vi "Switch Configure (3706).vi"(7 "Resistivity":T1, 8 "error in (no error)":errorcluster, 11 "VISA resource name in":refnum<visa-resource-name>) -> (0 "error out":errorcluster, 3 "VISA resource name out":refnum<visa-resource-name>)   [LabVIEW 2016, in "Hall Effect Library.lvlib"]
uses:
  Hall Effect Library.lvlib
  Public/Controls/Resisitivity.ctl
  Global Variables/Test Settings.vi
  <instrlib>/Keithley 3706/Keithley 3706.lvlib
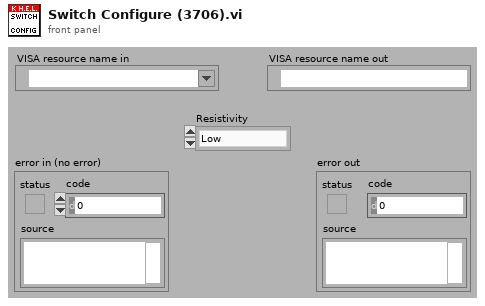
[diagram p1: front panel]
types:
  T1 = typedef "Hall Effect Library.lvlib/Resisitivity.ctl" = enum16{"Low", "High"}
  T2 = enum16{"BBM:Break Before Make", "MBB:Make Before Break", "OFF"}
  T3 = enum16{"None", "7052", "7053", "7054", "7056", "7057", "7058", "7059", "7061", "7062", "7063", "7064", "7065", "7066", "7067", "7152", "7153", "7154", "7156", "7158", "7164", "7166", "7168", "7169", "7402", "9990", "9991"}
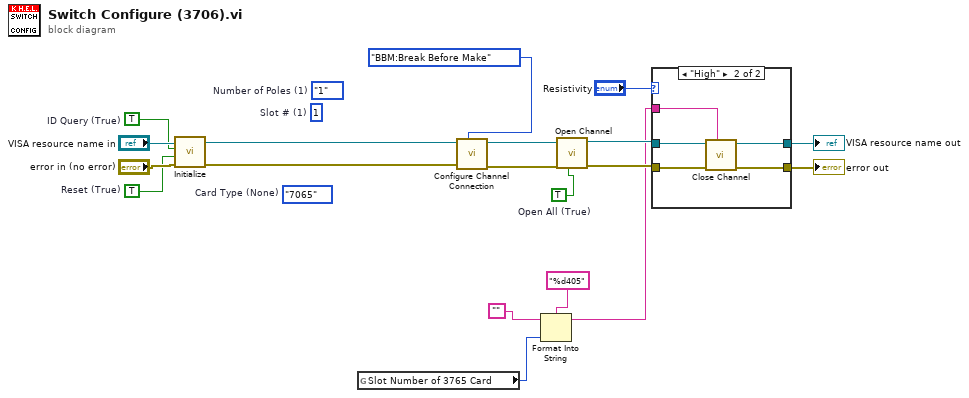
[diagram p0: block diagram]
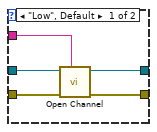
[diagram p2: hidden frame]
diagram:
  w9 = TRUE  # Open All (True)
  (unwired) enum16{"1", "2", "4"}."1"  # Number of Poles (1)
  (unwired) T3."7065"  # Card Type (None)
  w14 = TRUE  # Reset (True)
  w13 = TRUE  # ID Query (True)
  (unwired) u32 1  # Slot # (1)
  n1 = call <instrlib>:"Initialize.vi"("error in (no error)"="error in (no error)", "Reset (True)"=w14, "ID Query (True)"=w13, "VISA resource name"="VISA resource name in") -> ("error out"=w11:errorcluster, "VISA resource name out"=w12:refnum<visa-resource-name>)  [unwired: 6 in]
  n2 = global read "Test Settings.vi" "Slot Number of 3765 Card"() -> (w4:u32)
  n3 = call <instrlib>:"Configure Channel Connection.vi"("Channel Connect Rule"=T2."BBM:Break Before Make", "error in"=w11, "VISA resource name"=w12) -> ("error out"=w7:errorcluster, "VISA resource name out"=w8:refnum<visa-resource-name>)  [unwired: 7 in]
  n4 = Format Into String(format string="%d405", initial string="", w4) -> (resulting string=w1:string)  [unwired: 1 in, 1 out]
  n5 = call <instrlib>:"Open Channel.vi"("Open All (False)"=w9, "error in (no error)"=w7, "VISA resource name"=w8) -> ("error out"=w5:errorcluster, "VISA resource name out"=w6:refnum<visa-resource-name>)  [unwired: 7 in]
  n6 = case shown="\"High\"" "Resistivity" {
    tunnel: w1 -> [w24 w29]
    tunnel: w6 -> [w23 w28]
    tunnel: w5 -> [w22 w27]
    tunnel: [w20 w25] -> w17
    tunnel: [w21 w26] -> w18
    frame "Low", Default {
      n7 = call <instrlib>:"Open Channel.vi"("Channel List"=w24, "error in (no error)"=w22, "VISA resource name"=w23) -> ("error out"=w20:errorcluster, "VISA resource name out"=w21:refnum<visa-resource-name>)  [unwired: 7 in]
    }
    frame "High" {
      n8 = call <instrlib>:"Close Channel.vi"("Channel List"=w29, "error in (no error)"=w27, "VISA resource name"=w28) -> ("error out"=w25:errorcluster, "VISA resource name out"=w26:refnum<visa-resource-name>)  [unwired: 7 in]
    }
  }
  "error out" <- w17
  "VISA resource name out" <- w18
